vi "Relative or Abs Handler.vi"(10 "Set or Get":enum16{"Set", "Get"}(ring), 11 "Use Shortest Distance Relative?":bool=TRUE) -> (3 "Use Shortest Distance Relative? Out":bool)   [LabVIEW 2011, in "Pivot Drive.lvlib"]
uses:
  Pivot Drive.lvlib
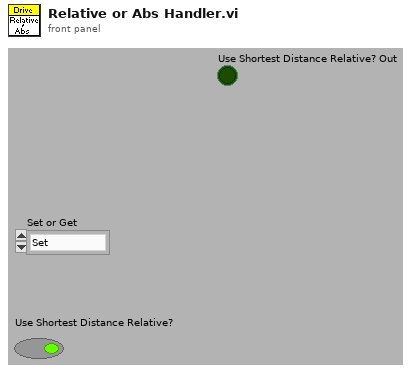
[diagram p1: front panel]
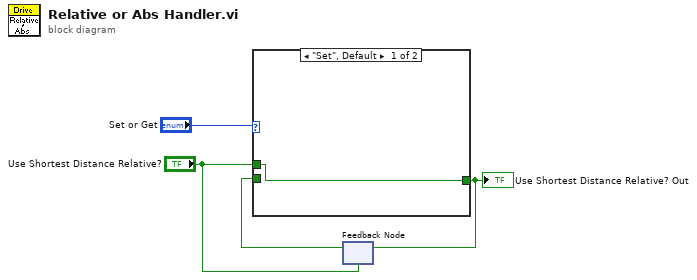
[diagram p0: block diagram]
diagram:
  n1 = feedback #1("Use Shortest Distance Relative?") -> (w3:bool)
  n2 = case shown="\"Set\", Default" "Set or Get" {
    tunnel: [w5 w6] -> w2
    tunnel: w3 -> [_ w6]
    tunnel: "Use Shortest Distance Relative?" -> [w5 _]
    frame "Set", Default {
    }
    frame "Get" {
    }
  }
  "Use Shortest Distance Relative? Out" <- w2
  n3 = feedback-in #1(w2) -> ()
